vi "Device Visualization.vi"(8 "error in (no error)":errorcluster, 9 "Device Name":string, 10 "Device #":string, 11 "Reference":refnum<vi>) -> (0 "error out":errorcluster)   [LabVIEW 2020, in "Retrieve and Visualize.lvclass"]
uses:
  Retrieve and Visualize.lvclass
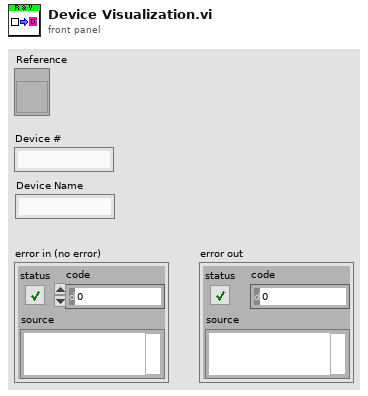
[diagram p1: front panel]
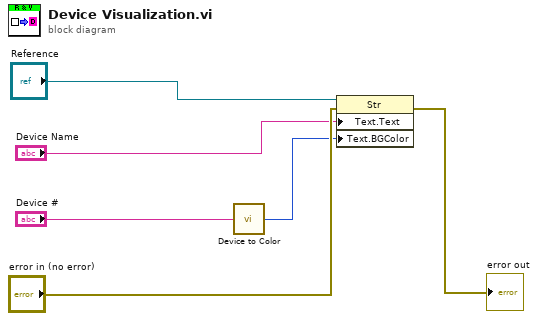
[diagram p0: block diagram]
diagram:
  n1 = call "Device to Color.vi"("Device #"="Device #") -> ("Color"=w2:u32)
  n2 = property on="Property Node" class="Str"(reference="Reference", error in="error in (no error)", "Text.Text"="Device Name", "Text.BGColor"=w2) -> (error out=→"error out":errorcluster)  [unwired: 1 out]
